vi "Index Riffle.vi"(9 "NRiffle":i32, 11 "N":i32) -> (2 "Riffled Indices":i32[](array[numeric]))   [LabVIEW 2015]
uses:
  <vilib>/Analysis/1siggen.llb/Riffle Array (I32) (obs 2012).vi
  <vilib>/Analysis/NI_AALBase.lvlib
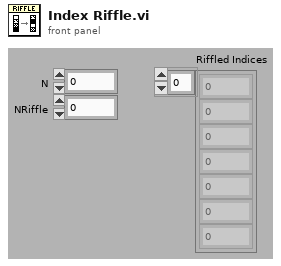
[diagram p1: front panel]
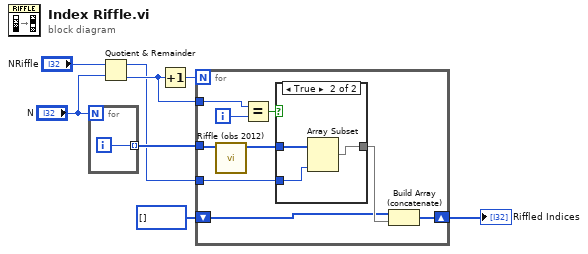
[diagram p0: block diagram]
diagram:
  n1 = for {
    N: "N" -> [_]
    tunnel: [w9] -> w5 mode=indexing
    i -> [w9]
  }
  n2 = Quotient & Remainder(x="NRiffle", y="N") -> (x-y*floor(x/y)=w2:i32, floor(x/y)=w4:i32)
  n3 = Increment(x=w4) -> (x+1=w6:i32)
  n4 = for {
    N: w6 -> [_]
    tunnel: w5 -> [w18]
    tunnel: w4 -> [w16]
    shift-right: [w12] -> w1
    shift-left: i32[] [] -> [w11]
    tunnel: w2 -> [w10]
    i -> [w17]
    n5 = call-poly <vilib>:"Riffle (obs 2012).vi"("X"=w18) -> ("Riffled {X}"=w14:i32[])  [unwired: 8 in, 2 out]
    n6 = Equal?(x=w16, y=w17) -> (x = y?=w15:bool)
    n7 = case shown="True" w15 {
      tunnel: w14 -> [w19 w22]
      tunnel: [w19 w21] -> w13
      tunnel: w10 -> [_ w20]
      frame False {
      }
      frame True {
        n8 = Array Subset(array=w22, length=w20) -> (w21:i32[])  [unwired: 1 in]
      }
    }
    n9 = Build Array (concatenate)(w11, w13) -> (w12:i32[])
  }
  "Riffled Indices" <- w1
